vi "Find Duplicate.vi"(10 "strings":string[](array[string])) -> (1 "index 1":i32, 2 "index 2":i32, 3 "duplicate exists":bool)   [LabVIEW 2014, in "tag bus configurable plugin module configuration.lvclass"]
uses:
  tag bus configurable plugin module configuration.lvclass
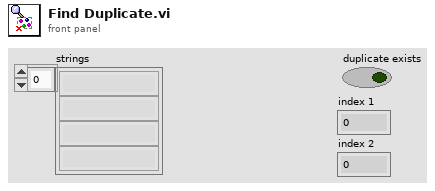
[diagram p1: front panel]
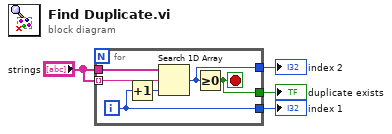
[diagram p0: block diagram]
diagram:
  n1 = for {
    tunnel: "strings" -> [w10]
    tunnel: "strings" -> [w9] mode=indexing
    tunnel: [w8] -> w2
    tunnel: [w6] -> w3
    tunnel: [w5] -> w4
    i -> [w6]
    stop <- w8 stop-if-true
    n2 = Increment(x=w6) -> (x+1=w7:i32)
    n3 = Search 1D Array(1D array=w10, element=w9, start index (0)=w7) -> (index of element=w5:i32)
    n4 = Greater Or Equal To 0?(x=w5) -> (x >= 0?=w8:bool)
  }
  "index 2" <- w4
  "index 1" <- w3
  "duplicate exists" <- w2
